vi "DELETE.vi"(8 "error in (no error)":errorcluster, 10 "relative URL":string, 11 "eLab in":refnum<class "PL eLabFTW Client.lvclass">) -> (0 "error out":errorcluster, 2 "response body":string, 3 "eLab out":refnum<class "PL eLabFTW Client.lvclass">)   [LabVIEW 2015, in "PL eLabFTW Client.lvclass"]
doc: "Performs DELETE request with the specified relative URL and returns the response body."
uses:
  PL eLabFTW Client.lvclass
  PL eLabFTW Client.lvclass/PL eLabFTW Client.ctl
  <vilib>/httpClient/LabVIEWHTTPClient.lvlib
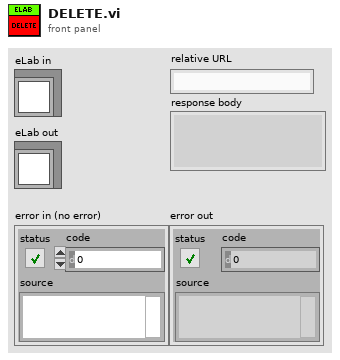
[diagram p1: front panel]
types:
  T1 = typedef "LabVIEWHTTPClient.lvlib/ClientHandle.ctl" = refnum<k1>
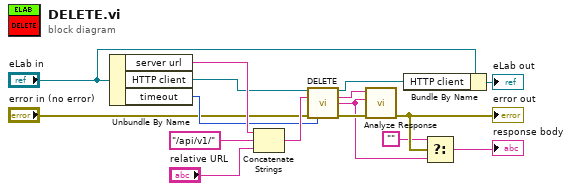
[diagram p0: block diagram]
diagram:
  n1 = Unbundle By Name("eLab in") -> ("server url"=w16:string, "HTTP client"=w4:T1, "timeout"=w13:i32)
  n2 = Concatenate Strings(w16, "/api/v1/" ("string"), "relative URL") -> (w14:string)
  n3 = call <vilib>:"DELETE.vi"("client handle"=w4, "url"=w14, "error in (no error)"="error in (no error)", "timeout (10000)"=w13) -> ("client handle out"=w1:T1, "headers"=w9:string, "body"=w7:string, "error out"=w10:errorcluster)  [unwired: 8 in]
  n4 = call "Analyze Response.vi"("error in (no error)"=w10, "body"=w7, "headers"=w9) -> ("error out"=w8:errorcluster)  [unwired: 8 in]
  "error out" <- w8
  n5 = Bundle By Name(cluster="eLab in", "HTTP client"=w1) -> (→"eLab out":refnum<class "PL eLabFTW Client.lvclass">)
  n6 = Select(t="", s=w8, f=w7) -> (s? t:f=→"response body":string)
